vi "Load Image (Path).vi"(8 "error in (no error)":errorcluster, 11 "Path In":path) -> (0 "error out":errorcluster, 2 "Image":T1, 3 "Path Out":path)   [LabVIEW 2020, in "G-Image.lvlib"]
doc: "Load an image file from disk and return it as a LabVIEW picture.\n\nSupported image types:\nPNG, JPEG, BMP, GIF, TGA, PSD, HDR, PIC, PNM\n\nWhen loading an animated GIF, only the first frame will be returned. Use <b>Load Animated GIF Image.vi</b> to read all frames."
uses:
  G-Image.lvlib
  <vilib>/picture/picture.llb/imagedata.ctl
  Private/Result To Error.vi
  <vilib>/Utility/error.llb/Error Cluster From Error Code.vi
  Private/Copy Image To Picture.vi
  <vilib>/picture/picture.llb/Create Mask By Alpha.vi
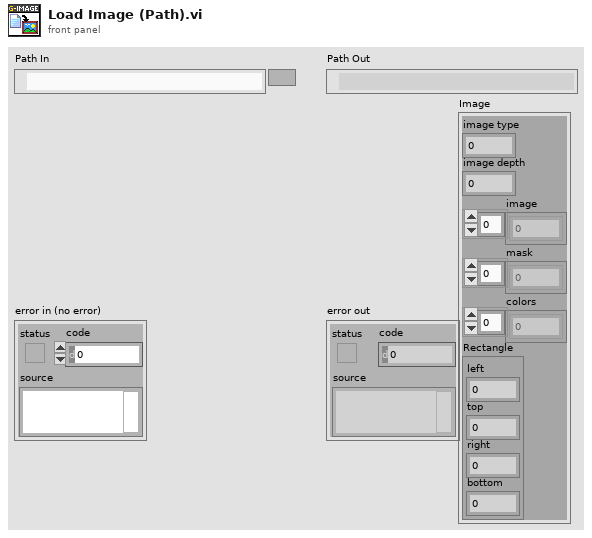
[diagram p1: front panel]
types:
  T1 = typedef "imagedata.ctl" = cluster{"image type":i32, "image depth":i32, "image":u8[], "mask":u8[], "colors":u32[], "Rectangle":cluster{"left":i16, "top":i16, "right":i16, "bottom":i16}}
  T2 = typedef "G-Image.lvlib/Extended Image.ctl" = cluster{"Image":T1, "Layers":i32, "Delays":i32[]}
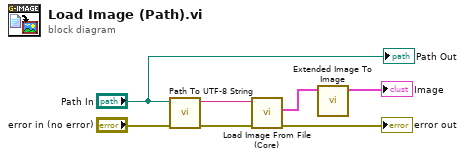
[diagram p0: block diagram]
diagram:
  n1 = call "Path To UTF-8 String.vi"("error in"="error in (no error)", "Path"="Path In") -> ("error out"=w3:errorcluster, "UTF-8 String"=w6:string)  [unwired: 8 in]
  n2 = call "Load Image From File (Core).vi"("error in (no error)"=w3, "Path In"=w6) -> ("error out"=→"error out":errorcluster, "Extended Image"=w1:T2)  [unwired: 7 in, 1 out]
  n3 = call "Extended Image To Image.vi"("Extended Image"=w1) -> ("Image"=→"Image":T1)  [unwired: 10 in]
  "Path Out" <- "Path In"
